vi "Open Device.vi"(8 "error in (no error)":errorcluster, 11 "DevState":T1={"Type"=41, "Index"=0, "DeviceOpen"=FALSE, "Ch0Start"=FALSE, "Ch1Start"=FALSE} {"Index" items=["0", "1", "2", "3", "4", "5", "6", "7", "8"]; "Type" items=["USBCANFD-200U"=41, "USBCANFD-100U"=42]}) -> (0 "error out":errorcluster, 3 "DevState out":T1={"Type"=41, "Index"=0, "DeviceOpen"=FALSE, "Ch0Start"=FALSE, "Ch1Start"=FALSE} {"Index" items=["0", "1", "2", "3", "4", "5", "6", "7", "8"]; "Type" items=["USBCANFD-200U"=41, "USBCANFD-100U"=42]})   [LabVIEW 2018, in "CAN FD.lvlib"]
uses:
  CAN FD.lvlib
  SubVI/zlgcan.lvlib
panel:
  # "e"
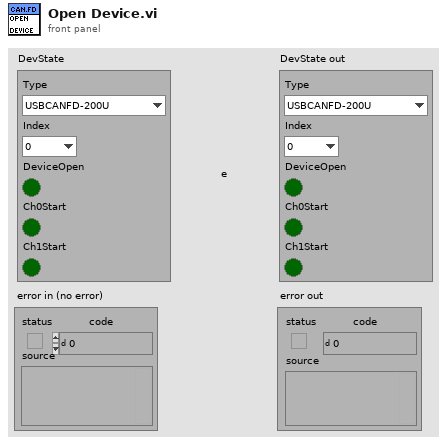
[diagram p1: front panel]
types:
  T1 = cluster{"Type":u32, "Index":u32, "DeviceOpen":bool, "Ch0Start":bool, "Ch1Start":bool}
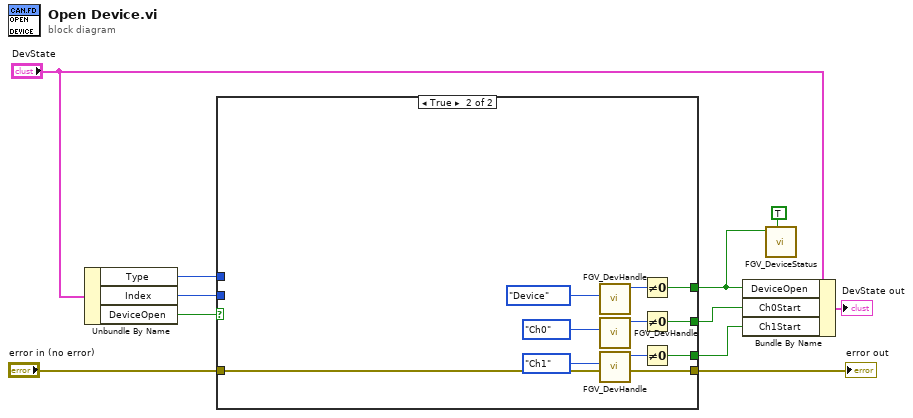
[diagram p0: block diagram]
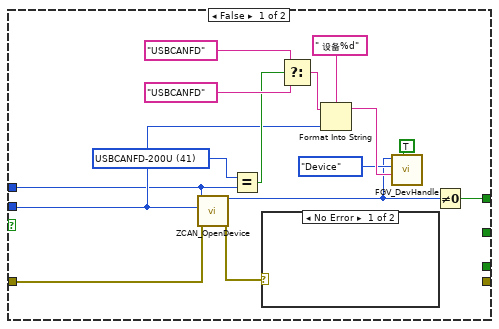
[diagram p2: hidden frame]
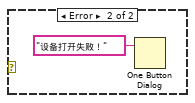
[diagram p3: hidden frame]
diagram:
  n1 = Unbundle By Name("DevState") -> ("Type"=w8:u32, "Index"=w7:u32, "DeviceOpen"=w11:bool)
  n2 = case shown="True" w11 {
    tunnel: "error in (no error)" -> [w15 w37]
    tunnel: [_ w37] -> w9
    tunnel: w8 -> [w16 _]
    tunnel: w7 -> [w17 _]
    tunnel: [w14 w34] -> w2
    tunnel: [_ w31] -> w4
    tunnel: [_ w28] -> w3
    frame False {
      w18 = u32 41 items=["USBCANFD-200U"=41, "USBCANFD-100U"=42] ("Type")
      n3 = call "ZCAN_OpenDevice.vi"("error in (no error)"=w15, "device_index"=w17, "device_type"=w16) -> ("error out"=w13:errorcluster, "DEVICE_HANDLE"=w12:u64)  [unwired: 7 in]
      n4 = Equal?(x=w18, y=w16) -> (x = y?=w21:bool)
      n5 = case shown="No Error" w13 {
        frame No Error {
        }
        frame Error {
          n6 = One Button Dialog(message="设备打开失败！" ("消息")) -> ()  [unwired: 1 in, 1 out]
        }
      }
      n7 = Select(t="USBCANFD", s=w21, f="USBCANFD") -> (s? t:f=w24:string)
      n8 = Format Into String(format string=" 设备%d" ("格式字符串"), initial string=w24, w17) -> (resulting string=w26:string)  [unwired: 1 in, 1 out]
      n9 = call "FGV_DevHandle.vi"("Set"=TRUE, "Name"=w26, "Type"=enum16{"Device", "Ch0", "Ch1"}."Device", "handle"=w12) -> ()  [unwired: 5 in, 3 out]
      n10 = Not Equal To 0?(x=w12) -> (x != 0?=w14:bool)
    }
    frame True {
      n11 = call "FGV_DevHandle.vi"("Type"=enum16{"Device", "Ch0", "Ch1"}."Device") -> ("handle out"=w35:u64)  [unwired: 8 in, 2 out]
      n12 = call "FGV_DevHandle.vi"("Type"=enum16{"Device", "Ch0", "Ch1"}."Ch0") -> ("handle out"=w33:u64)  [unwired: 8 in, 2 out]
      n13 = call "FGV_DevHandle.vi"("Type"=enum16{"Device", "Ch0", "Ch1"}."Ch1") -> ("handle out"=w29:u64)  [unwired: 8 in, 2 out]
      n14 = Not Equal To 0?(x=w35) -> (x != 0?=w34:bool)
      n15 = Not Equal To 0?(x=w33) -> (x != 0?=w31:bool)
      n16 = Not Equal To 0?(x=w29) -> (x != 0?=w28:bool)
    }
  }
  "error out" <- w9
  n17 = Bundle By Name(cluster="DevState", "DeviceOpen"=w2, "Ch0Start"=w4, "Ch1Start"=w3) -> (→"DevState out":T1)
  n18 = call "FGV_DeviceStatus.vi"("Set"=TRUE, "Open"=w2) -> ()  [unwired: 8 in, 2 out]
